vi "WAV_Chunks.vi"(11 "contents":string) -> (3 "Chunks":T1(array[cluster]))   [LabVIEW 2022 SP3]
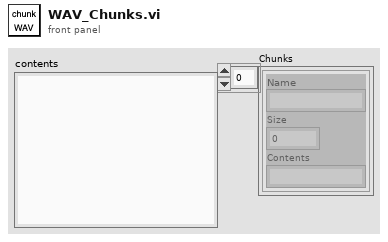
[diagram p1: front panel]
types:
  T1 = cluster{"Name":string, "Size":u32, "Contents":string}[]
  T2 = enum16{"big-endian, network order", "native, host order", "little-endian"}
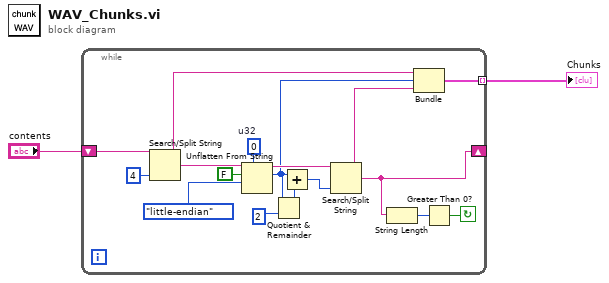
[diagram p0: block diagram]
diagram:
  n1 = while {
    shift-right: [w13] -> _
    shift-left: "contents" -> [w19]
    tunnel: [w10] -> w2 mode=indexing
    stop <- w5 continue-if-true
    w16 = u32 0  # u32
    n2 = Search/Split String(string=w19, offset (0)=4) -> (substring before match=w11:string, match + rest of string=w6:string)  [unwired: 1 in, 1 out]
    n3 = Unflatten From String(type=w16, binary string=w6, data includes array or string size? (T)=FALSE, byte order (0:big-endian, network order)=T2."little-endian") -> (rest of the binary string=w14:string, value=w3:u32)  [unwired: 1 in, 1 out]
    n4 = Quotient & Remainder(x=w3, y=u32 2 ("count")) -> (x-y*floor(x/y)=w8:u32)  [unwired: 1 out]
    n5 = Add(x=w3, y=w8) -> (x+y=w7:u32)
    n6 = Search/Split String(string=w14, offset (0)=w7) -> (substring before match=w4:string, match + rest of string=w13:string)  [unwired: 1 in, 1 out]
    n7 = String Length(string=w13) -> (length=w12:i32)
    n8 = Bundle("contents"=w11, "u32"=w3, w4) -> (w10:cluster{"contents":string, "u32":u32, string})  [unwired: 1 in]
    n9 = Greater Than 0?(x=w12) -> (x > 0?=w5:bool)
  }
  "Chunks" <- w2
